vi "Graham Scan 3-point Cross Product.vi"(1 "C":T1, 2 "B":T1, 3 "A":T1) -> (0 "|| AB X AC ||":i32)   [LabVIEW 2018]
uses:
  Graham Scan Point.ctl
  <vilib>/Analysis/NI_AALPro.lvlib
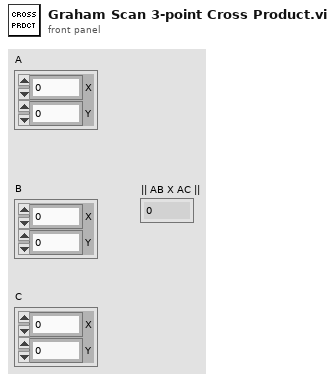
[diagram p1: front panel]
types:
  T1 = typedef "Graham Scan Point.ctl" = cluster{"X":i32, "Y":i32}
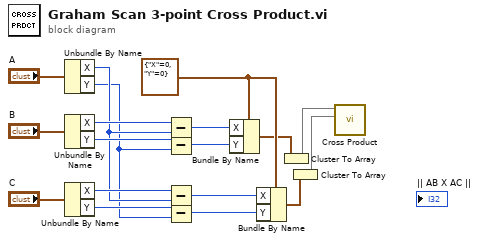
[diagram p0: block diagram]
diagram:
  w7 = T1 {"X"=0, "Y"=0} ("Point")
  n1 = Unbundle By Name("A") -> ("X"=w12:i32, "Y"=w10:i32)
  n2 = Unbundle By Name("B") -> ("X"=w15:i32, "Y"=w14:i32)
  n3 = Unbundle By Name("C") -> ("X"=w13:i32, "Y"=w11:i32)
  n4 = Subtract(x=w15, y=w12) -> (x-y=w9:i32)
  n5 = Subtract(x=w14, y=w10) -> (x-y=w8:i32)
  n6 = Subtract(x=w13, y=w12) -> (x-y=w6:i32)
  n7 = Subtract(x=w11, y=w10) -> (x-y=w5:i32)
  n8 = Bundle By Name(cluster=w7, "X"=w9, "Y"=w8) -> (w4:T1)
  n9 = Bundle By Name(cluster=w7, "X"=w6, "Y"=w5) -> (w3:T1)
  n10 = Cluster To Array(cluster=w4) -> (array=w2:i32[])
  n11 = Cluster To Array(cluster=w3) -> (array=w1:i32[])
  n12 = call <vilib>:"Cross Product.vi"("B Vector"=w1, "A Vector"=w2) -> ()  [unwired: 8 in, 2 out]
